vi "ExecuteXML.vi"(8 "error in (no error)":errorcluster, 11 "Auto File Path":path=path "C:/Users/Bendethic/Desktop/AutoRoutineCreator/AutoFiles/1A.txt") -> (0 "error out (no error)":errorcluster)   [LabVIEW 2017]
uses:
  <resource>/objmgr/DOMUserDefRef.rc
  <vilib>/xml/NI_XML.lvlib
  <vilib>/xml/Close Reference(Node).vi
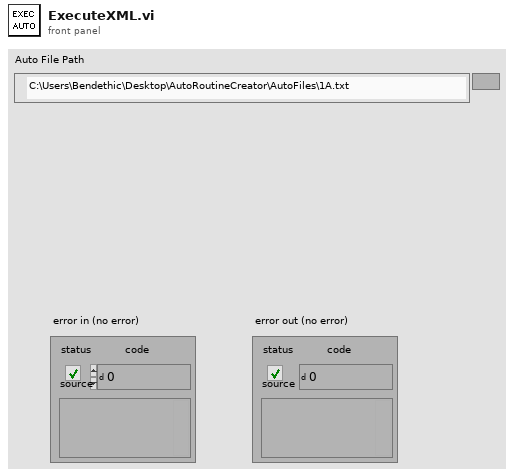
[diagram p1: front panel]
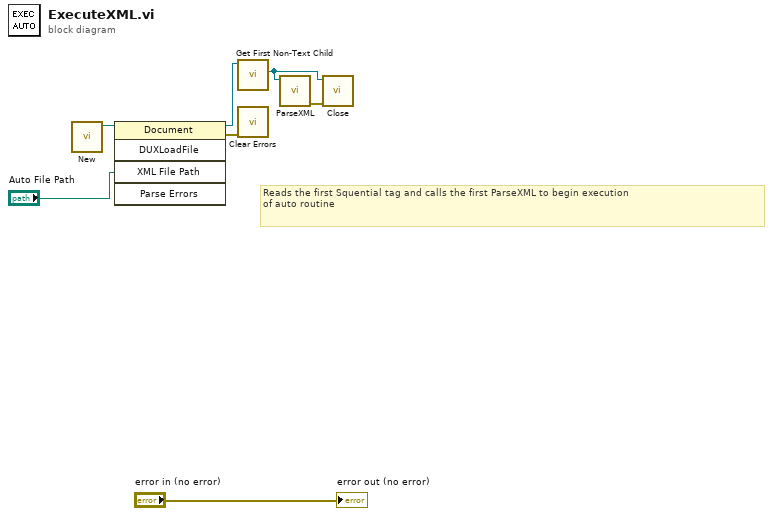
[diagram p0: block diagram]
diagram:
  # "Reads the first Squential tag and calls the first ParseXML to begin execution\nof auto routine"
  n1 = call <vilib>:"New.vi"() -> ("DOM document out"=w6:refnum<k20>)  [unwired: 8 in, 1 out]
  n2 = invoke class="Document" method="DUXLoadFile"(reference=w6, "XML File Path"="Auto File Path") -> (reference out=w4:refnum<k20>, error out=w5:errorcluster)  [unwired: 3 in, 3 out]
  n3 = call <vilib>:"Get First Non-Text Child.vi"("node in"=w4) -> ("child node"=w2:refnum<k20>)  [unwired: 7 in, 3 out]
  n4 = call <vilib>:"Clear Errors.vi"("error in (no error)"=w5) -> ()  [unwired: 5 in, 2 out]
  n5 = call "ParseXML.vi"("Node"=w2) -> ("error out"=w3:errorcluster)  [unwired: 10 in]
  n6 = call-poly <vilib>:"Close.vi"("error in (no error)"=w3, "node"=w2) -> ()  [unwired: 7 in, 1 out]
  "error out (no error)" <- "error in (no error)"
